vi "Conditions.vi"(1 "Set current":bool, 2 "New condition code":i32) -> (16 "Condition code":i32, 18 "Current condition":T1={"Type"=enum."Start", "Task"=2, "Code"="", "Duration"=0.0, "Prompts"=2, "Mode controls"={"Hold"=FALSE, "Cancellation"=FALSE, "Goal filter"=FALSE, "Trigger"=FALSE}, "Variable"=FALSE, "Hold"=FALSE})   [LabVIEW 2012]
uses:
  condition_tab.ctl
  trial_condition.ctl
  testing/mode_conrols.ctl
panel:
  in  "Current condition code":i32
  in  "Condition table":T3[](array[typedef])=[{"Type"=enum."Start", "Task"=0, "Duration"=0.0, "Prompts"=0, "Cancellation"=TRUE, "Goal filter"=TRUE, "Variable"=FALSE, "Hold"=FALSE}, {"Type"=enum."Normal", "Task"=0, "Duration"=20.0, "Prompts"=1, "Cancellation"=FALSE, "Goal filter"=FALSE, "Variable"=FALSE, "Hold"=FALSE}, {"Type"=enum."Normal", "Task"=1, "Duration"=30.0, "Prompts"=1, "Cancellation"=FALSE, "Goal filter"=FALSE, "Variable"=TRUE, "Hold"=FALSE}, {"Type"=enum."Normal", "Task"=0, "Duration"=20.0, "Prompts"=1, "Cancellation"=TRUE, "Goal filter"=TRUE, "Variable"=FALSE, "Hold"=TRUE}, {"Type"=enum."Normal", "Task"=1, "Duration"=30.0, "Prompts"=1, "Cancellation"=TRUE, "Goal filter"=TRUE, "Variable"=TRUE, "Hold"=FALSE}, {"Type"=enum."Normal", "Task"=0, "Duration"=20.0, "Prompts"=1, "Cancellation"=TRUE, "Goal filter"=TRUE, "Variable"=FALSE, "Hold"=FALSE}, {"Type"=enum."Undefined", "Task"=0, "Duration"=30.0, "Prompts"=1, "Cancellation"=FALSE, "Goal filter"=FALSE, "Variable"=FALSE, "Hold"=FALSE}, {"Type"=enum."Undefined", "Task"=2, "Duration"=60.0, "Prompts"=4, "Cancellation"=TRUE, "Goal filter"=TRUE, "Variable"=FALSE, "Hold"=FALSE}, {"Type"=enum."Undefined", "Task"=2, "Duration"=60.0, "Prompts"=4, "Cancellation"=TRUE, "Goal filter"=FALSE, "Variable"=FALSE, "Hold"=FALSE}, {"Type"=enum."Undefined", "Task"=2, "Duration"=60.0, "Prompts"=4, "Cancellation"=FALSE, "Goal filter"=TRUE, "Variable"=FALSE, "Hold"=FALSE}, {"Type"=enum."Rest", "Task"=0, "Duration"=240.0, "Prompts"=0, "Cancellation"=FALSE, "Goal filter"=TRUE, "Variable"=FALSE, "Hold"=FALSE}, {"Type"=enum."Undefined", "Task"=3, "Duration"=180.0, "Prompts"=1, "Cancellation"=TRUE, "Goal filter"=TRUE, "Variable"=TRUE, "Hold"=FALSE}, {"Type"=enum."Undefined", "Task"=3, "Duration"=180.0, "Prompts"=1, "Cancellation"=FALSE, "Goal filter"=TRUE, "Variable"=TRUE, "Hold"=FALSE}, {"Type"=enum."Undefined", "Task"=0, "Duration"=0.0, "Prompts"=0, "Cancellation"=FALSE, "Goal filter"=TRUE, "Variable"=FALSE, "Hold"=FALSE}, {"Type"=enum."Undefined", "Task"=0, "Duration"=0.0, "Prompts"=0, "Cancellation"=FALSE, "Goal filter"=TRUE, "Variable"=FALSE, "Hold"=FALSE}, {"Type"=enum."Undefined", "Task"=0, "Duration"=0.0, "Prompts"=0, "Cancellation"=FALSE, "Goal filter"=TRUE, "Variable"=FALSE, "Hold"=FALSE}, {"Type"=enum."Undefined", "Task"=0, "Duration"=0.0, "Prompts"=0, "Cancellation"=FALSE, "Goal filter"=TRUE, "Variable"=FALSE, "Hold"=FALSE}, {"Type"=enum."Undefined", "Task"=0, "Duration"=0.0, "Prompts"=0, "Cancellation"=FALSE, "Goal filter"=TRUE, "Variable"=FALSE, "Hold"=FALSE}, {"Type"=enum."Undefined", "Task"=0, "Duration"=0.0, "Prompts"=0, "Cancellation"=FALSE, "Goal filter"=TRUE, "Variable"=FALSE, "Hold"=FALSE}, {"Type"=enum."Undefined", "Task"=0, "Duration"=0.0, "Prompts"=0, "Cancellation"=FALSE, "Goal filter"=TRUE, "Variable"=FALSE, "Hold"=FALSE}, {"Type"=enum."Undefined", "Task"=0, "Duration"=0.0, "Prompts"=0, "Cancellation"=FALSE, "Goal filter"=TRUE, "Variable"=FALSE, "Hold"=FALSE}, {"Type"=enum."Undefined", "Task"=0, "Duration"=0.0, "Prompts"=0, "Cancellation"=FALSE, "Goal filter"=TRUE, "Variable"=FALSE, "Hold"=FALSE}, {"Type"=enum."Undefined", "Task"=0, "Duration"=0.0, "Prompts"=0, "Cancellation"=FALSE, "Goal filter"=TRUE, "Variable"=FALSE, "Hold"=FALSE}, {"Type"=enum."Undefined", "Task"=0, "Duration"=0.0, "Prompts"=0, "Cancellation"=FALSE, "Goal filter"=TRUE, "Variable"=FALSE, "Hold"=FALSE}, {"Type"=enum."Undefined", "Task"=0, "Duration"=0.0, "Prompts"=0, "Cancellation"=FALSE, "Goal filter"=TRUE, "Variable"=FALSE, "Hold"=FALSE}, {"Type"=enum."Undefined", "Task"=0, "Duration"=0.0, "Prompts"=0, "Cancellation"=FALSE, "Goal filter"=TRUE, "Variable"=FALSE, "Hold"=FALSE}, {"Type"=enum."Undefined", "Task"=0, "Duration"=0.0, "Prompts"=0, "Cancellation"=FALSE, "Goal filter"=TRUE, "Variable"=FALSE, "Hold"=FALSE}, {"Type"=enum."Undefined", "Task"=0, "Duration"=0.0, "Prompts"=0, "Cancellation"=FALSE, "Goal filter"=TRUE, "Variable"=FALSE, "Hold"=FALSE}, {"Type"=enum."Undefined", "Task"=0, "Duration"=0.0, "Prompts"=0, "Cancellation"=FALSE, "Goal filter"=TRUE, "Variable"=FALSE, "Hold"=FALSE}, {"Type"=enum."Undefined", "Task"=0, "Duration"=0.0, "Prompts"=0, "Cancellation"=FALSE, "Goal filter"=TRUE, "Variable"=FALSE, "Hold"=FALSE}, {"Type"=enum."Undefined", "Task"=0, "Duration"=0.0, "Prompts"=0, "Cancellation"=FALSE, "Goal filter"=TRUE, "Variable"=FALSE, "Hold"=FALSE}, {"Type"=enum."Done", "Task"=0, "Duration"=0.0, "Prompts"=0, "Cancellation"=TRUE, "Goal filter"=TRUE, "Variable"=FALSE, "Hold"=FALSE}]
  # "Locals:"
  # "This lookup table defines the trial conditions, mapping the numeric condition code to the corresponding settings.  Conditions 0 and 31 are special, representing initial and final condition."
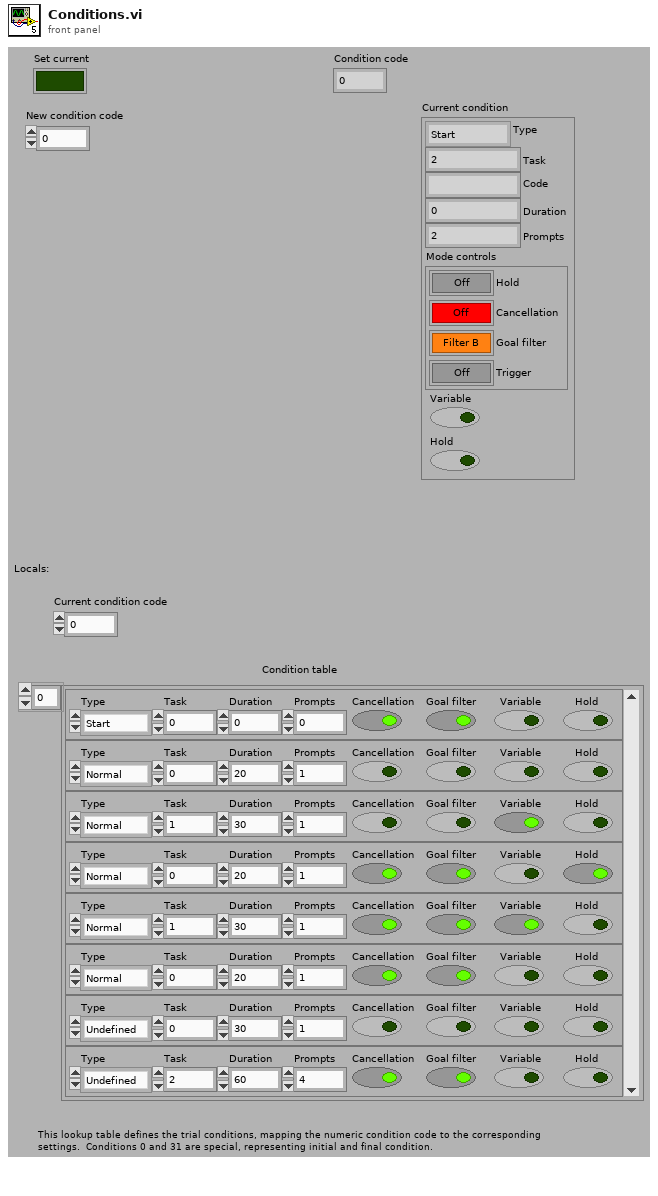
[diagram p1: front panel]
types:
  T1 = typedef "trial_condition.ctl" = cluster{"Type":enum16{"Undefined", "Start", "Normal", "Rest", "Done"}, "Task":u16, "Code":string, "Duration":dbl, "Prompts":u16, "Mode controls":T2, "Variable":bool, "Hold":bool}
  T2 = typedef "mode_conrols.ctl" = cluster{"Hold":bool, "Cancellation":bool, "Goal filter":bool, "Trigger":bool}
  T3 = typedef "condition_tab.ctl" = cluster{"Type":enum16{"Undefined", "Start", "Normal", "Rest", "Done"}, "Task":u16, "Duration":dbl, "Prompts":u16, "Cancellation":bool, "Goal filter":bool, "Variable":bool, "Hold":bool}
  T4 = enum16{"Undefined", "Start", "Normal", "Rest", "Done"}
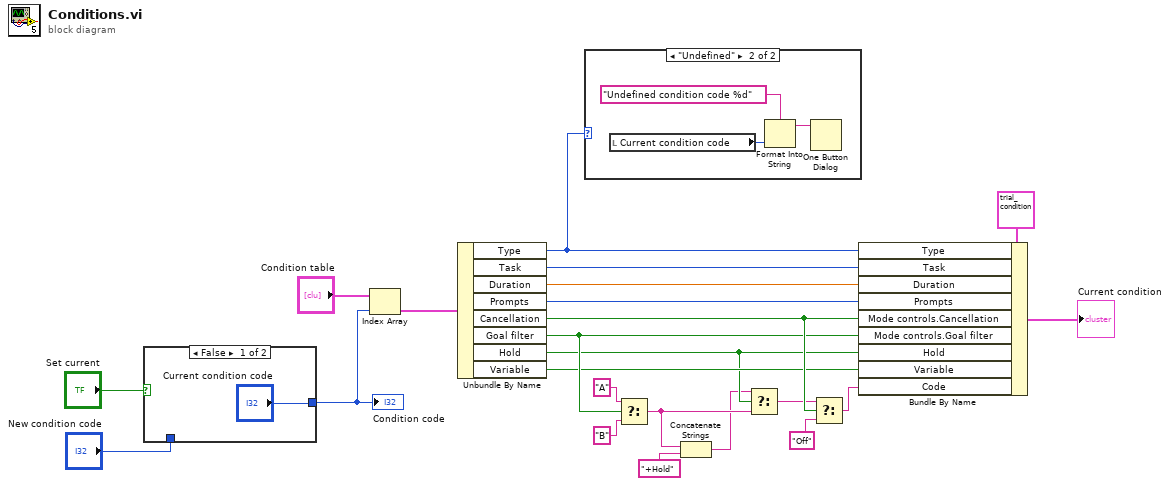
[diagram p0: block diagram]
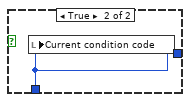
[diagram p3: hidden frame]
diagram:
  n1 = case shown="False" "Set current" {
    tunnel: "New condition code" -> [_ w25]
    tunnel: ["Current condition code" w25] -> w20
    frame False {
    }
    frame True {
      n2 = local write "Current condition code"(w25) -> ()
    }
  }
  "Condition code" <- w20
  n3 = Index Array(array="Condition table", index=w20) -> (element=w12:T3)
  n4 = Unbundle By Name(w12) -> ("Type"=w6:T4, "Task"=w19:u16, "Duration"=w18:dbl, "Prompts"=w11:u16, "Cancellation"=w15:bool, "Goal filter"=w10:bool, "Hold"=w5:bool, "Variable"=w7:bool)
  n5 = case shown="\"Undefined\"" w6 {
    frame "Start", Default {
    }
    frame "Undefined" {
      n6 = local read "Current condition code"() -> (w27:i32)
      n7 = Format Into String(format string="Undefined condition code %d", w27) -> (resulting string=w28:string)  [unwired: 2 in, 1 out]
      n8 = One Button Dialog(message=w28) -> ()  [unwired: 2 out]
    }
  }
  n9 = Select(t="A" ("f"), s=w10, f="B") -> (s? t:f=w4:string)
  n10 = Concatenate Strings(w4, "+Hold" ("string")) -> (w2:string)
  n11 = Select(t=w2, s=w5, f=w4) -> (s? t:f=w1:string)
  n12 = Select(t=w1, s=w15, f="Off") -> (s? t:f=w14:string)
  n13 = Bundle By Name(cluster=T1 {"Type"=enum."Start", "Task"=2, "Code"="", "Duration"=0.0, "Prompts"=0, "Mode controls"={"Hold"=FALSE, "Cancellation"=FALSE, "Goal filter"=FALSE, "Trigger"=FALSE}, "Variable"=FALSE, "Hold"=FALSE} ("Current condition"), "Type"=w6, "Task"=w19, "Duration"=w18, "Prompts"=w11, "Mode controls.Cancellation"=w15, "Mode controls.Goal filter"=w10, "Hold"=w5, "Variable"=w7, "Code"=w14) -> (→"Current condition":T1)
